vi "Read Digital Input Phase Noise.vi"(0 "VISA resource name":refnum<visa-resource-name>, 1 "Samples Count (1)":u32=1, 5 "Start Frequency (1 Hz)":dbl=1.0, 7 "Stop Frequency (1 Hz)":dbl=1.0, 11 "error in (no error)":errorcluster) -> (3 "Actual Level Amplitude":dbl format="%.8e", 4 "VISA resource name out":refnum<visa-resource-name>, 6 "Actual Start Frequency":dbl format="%.8e", 8 "Actual Stop Frequency":dbl format="%.8e", 14 "Theoretical Phase Noise Amplitude":dbl[](array[numeric]) format="%.8e", 15 "error out":errorcluster)   [LabVIEW 2018, in "Agilent PSG MXG Series.lvlib"]
doc: "Fetches the digital input phase noise measurements.\n\n<b>Note:</b>\nIt is applicable for N5172B/82B with <b>Option 004</b> only."
uses:
  Agilent PSG MXG Series.lvlib
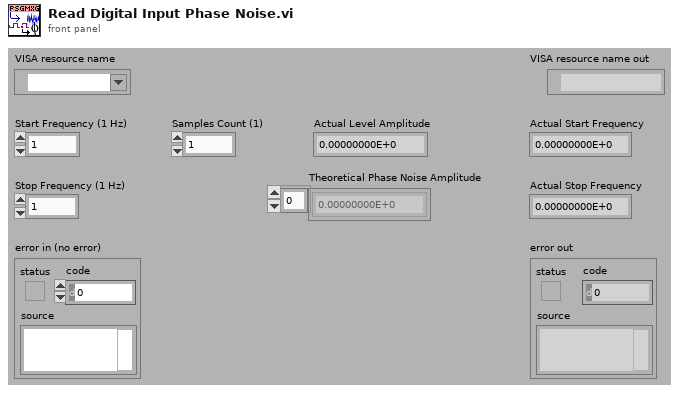
[diagram p1: front panel]
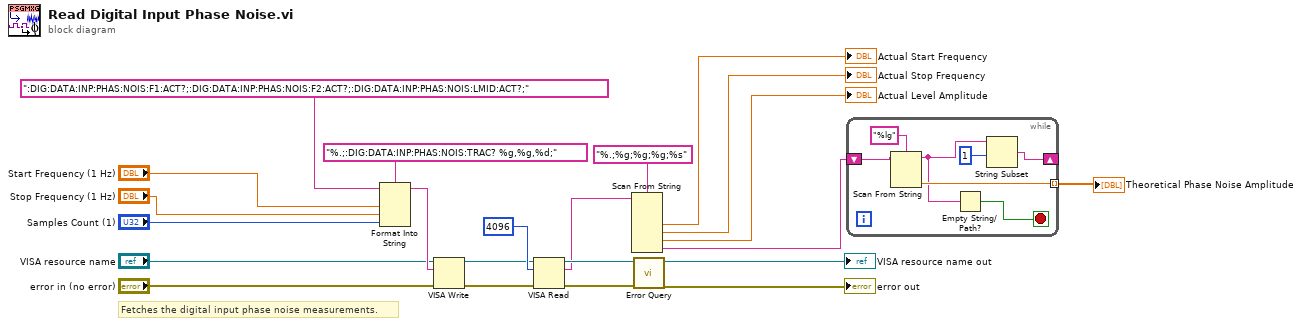
[diagram p0: block diagram]
diagram:
  # "Fetches the digital input phase noise measurements."
  n1 = Format Into String(format string="%.;:DIG:DATA:INP:PHAS:NOIS:TRAC? %g,%g,%d;", initial string=":DIG:DATA:INP:PHAS:NOIS:F1:ACT?;:DIG:DATA:INP:PHAS:NOIS:F2:ACT?;:DIG:DATA:INP:PHAS:NOIS:LMID:ACT?;", "Start Frequency (1 Hz)", "Stop Frequency (1 Hz)", "Samples Count (1)") -> (resulting string=w17:string)  [unwired: 1 in, 1 out]
  n2 = VISA Write(VISA resource name="VISA resource name", write buffer=w17, error in (no error)="error in (no error)") -> (VISA resource name out=w13:refnum<visa-resource-name>, error out=w12:errorcluster)  [unwired: 1 out]
  n3 = VISA Read(VISA resource name=w13, byte count=u32 4096, error in (no error)=w12) -> (VISA resource name out=w11:refnum<visa-resource-name>, read buffer=w7:string, error out=w10:errorcluster)  [unwired: 1 out]
  n4 = Scan From String(format string="%.;%g;%g;%g;%s", input string=w7) -> (output 1=→"Actual Start Frequency":dbl, output 2=→"Actual Stop Frequency":dbl, output 3=→"Actual Level Amplitude":dbl, output 4=w1:string)  [unwired: 6 in, 3 out]
  n5 = call "Error Query.vi"("error in (no error)"=w10, "VISA resource name"=w11) -> ("error out"=→"error out":errorcluster, "VISA resource name out"=→"VISA resource name out":refnum<visa-resource-name>)  [unwired: 6 in, 2 out]
  n6 = while {
    shift-right: [w25] -> _
    shift-left: w1 -> [w29]
    tunnel: [w27] -> w2 mode=indexing
    stop <- w23 stop-if-true
    n7 = Scan From String(format string="%lg", input string=w29) -> (remaining string=w24:string, output 1=w27:dbl)  [unwired: 3 in, 2 out]
    n8 = Empty String/Path?(string/path=w24) -> (empty?=w23:bool)
    n9 = String Subset(string=w24, offset (0)=1) -> (substring=w25:string)  [unwired: 1 in]
  }
  "Theoretical Phase Noise Amplitude" <- w2
